vi "Get Depth Frame.vi"(8 "error in (no error)":errorcluster, 11 "Kinect Session in":refnum<class "Kinect Session.lvclass">) -> (0 "error out":errorcluster, 1 "Grayscale depth image":T1, 2 "Depth Frame":T1(plugin-control), 3 "Kinect Session out":refnum<class "Kinect Session.lvclass">, 4 "Pixel depth array":i16[][](array[numeric]))   [LabVIEW 2014, in "Kinect Library.lvlib"]
doc: "This VI will retrieve the latest depth image. If this function is called too frequently, it can return an error. If the function is called too sparsely, nothing bad will happen."
uses:
  Kinect Library.lvlib
  Kinect Session Class/Kinect Session.lvclass
  <vilib>/vision/Image Controls.llb/IMAQ Image.ctl
  Microsoft.Kinect
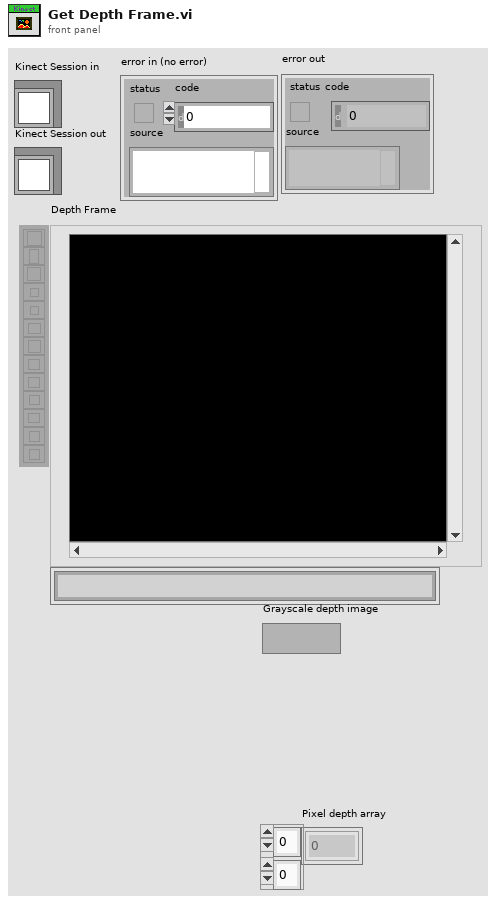
[diagram p1: front panel]
types:
  T1 = typedef "IMAQ Image.ctl" = refnum<image>
  T2 = typedef "Image Type" = u32
  T3 = cluster{"FramePixelDataLength":i32, "FrameWidth":i32, "FrameHeight":i32}
  T4 = cluster{"status":bool, "code":bool, "source":bool}
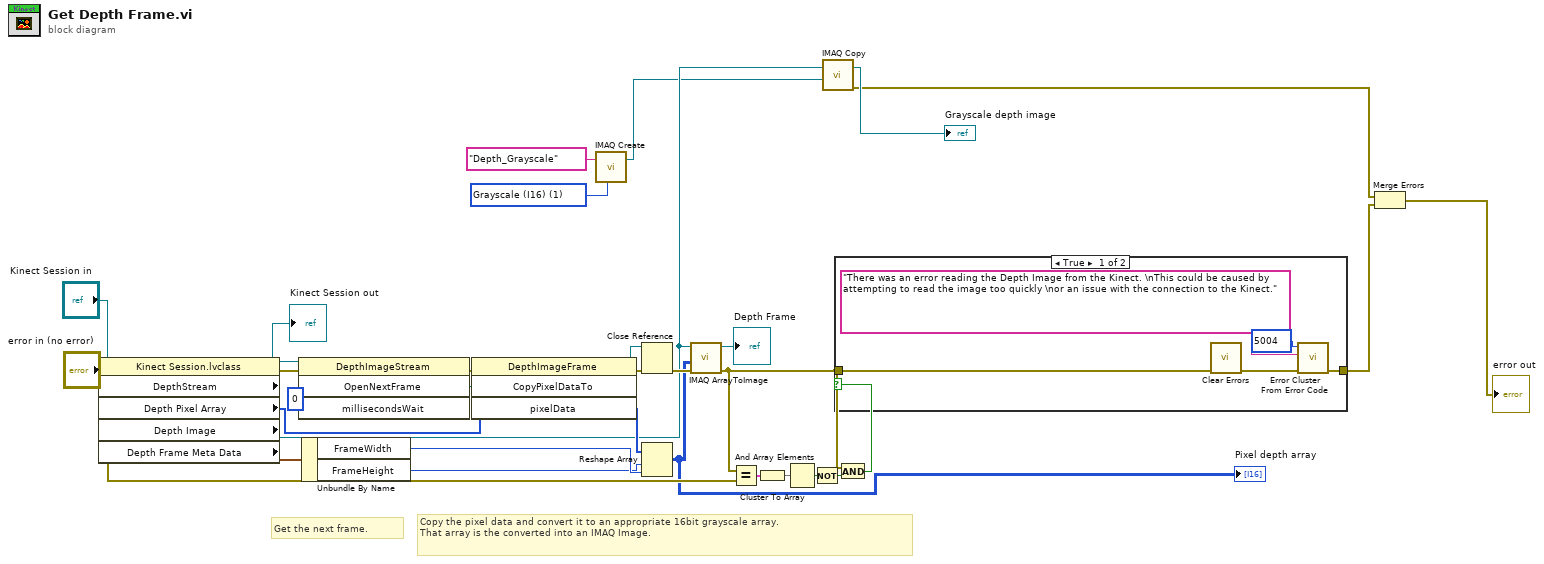
[diagram p0: block diagram]
diagram:
  w8 = T2 1 items=["Grayscale (U8)", "Grayscale (I16)", "Grayscale (SGL)", "Complex (CSG)", "RGB (U32)", "HSL (U32)", "RGB (U64)", "Grayscale (U16)"] ("Image Type")
  # "Copy the pixel data and convert it to an appropriate 16bit grayscale array.\nThat array is the converted into an IMAQ Image."
  # "Get the next frame."
  n1 = property class="Kinect Session.lvclass"(reference="Kinect Session in", error in="error in (no error)") -> (reference out=→"Kinect Session out":refnum<class "Kinect Session.lvclass">, error out=w19:errorcluster, "DepthStream"=w30:refnum<k24>, "Depth Pixel Array"=w27:i16[], "Depth Image"=w3:T1, "Depth Frame Meta Data"=w25:T3)
  n2 = invoke class="DepthImageStream" method="OpenNextFrame"(reference=w30, error in=w19, "millisecondsWait"=0) -> (error out=w21:errorcluster, "OpenNextFrame"=w28:refnum<k24>)  [unwired: 1 in, 2 out]
  n3 = Unbundle By Name(w25) -> ("FrameWidth"=w24:i32, "FrameHeight"=w23:i32)
  n4 = invoke class="DepthImageFrame" method="CopyPixelDataTo"(reference=w28, error in=w21, "pixelData"=w27) -> (reference out=w22:refnum<k24>, error out=w20:errorcluster, "pixelData"=w26:i16[])  [unwired: 1 in, 1 out]
  n5 = call "IMAQ Create"("Image Name"="Depth_Grayscale", "Image Type"=w8) -> ("New Image"=w2:T1)  [unwired: 3 in, 1 out]
  n6 = Close Reference(reference=w22, error in (no error)=w20) -> (error out=w18:errorcluster)
  n7 = Reshape Array(w26, w23, w24) -> (w10:i16[][])
  "Pixel depth array" <- w10
  n8 = call "IMAQ ArrayToImage"("error in (no error)"=w18, "Image Pixels (I16)"=w10, "Image"=w3) -> ("error out"=w14:errorcluster, "Image Out"=→"Depth Frame":T1)  [unwired: 7 in]
  n9 = Equal?(x=w14, y="error in (no error)") -> (x = y?=w17:T4)
  n10 = Cluster To Array(cluster=w17) -> (array=w16:bool[])
  n11 = And Array Elements(Boolean array=w16) -> (logical AND=w11:bool)
  n12 = Not(x=w11) -> (.not. x?=w15:bool)
  n13 = call "IMAQ Copy"("Image Dst"=w2, "Image Src"=w3) -> ("error out"=w1:errorcluster, "Image Dst Out"=→"Grayscale depth image":T1)  [unwired: 4 in]
  n14 = And(x=w14, y=w15) -> (x .and. y?=w13:bool)
  n15 = case shown="True" w13 {
    tunnel: [w37 w38] -> w7
    tunnel: w14 -> [w34 w38]
    frame True {
      n16 = call <vilib>:"Clear Errors.vi"("error in (no error)"=w34) -> ("error out"=w33:errorcluster)  [unwired: 5 in, 1 out]
      n17 = call <vilib>:"Error Cluster From Error Code.vi"("error in (no error)"=w33, "error message (\"\")"="There was an error reading the Depth Image from the Kinect. \nThis could be caused by attempting to read the image too quickly \nor an issue with the connection to the Kinect." ("error message (\"\")"), "error code (0)"=5004) -> ("error out"=w37:errorcluster)  [unwired: 6 in]
    }
    frame False {
    }
  }
  n18 = Merge Errors(w1, w7) -> (→"error out":errorcluster)
